vi "PELLETID.vi"(0 "NXT/EV3":T1) -> (6 "Marble ID#":i32, 7 "NXT/EV3 2":T1)   [LabVIEW 2016]
uses:
  <vilib>/NXT/Subs/LVHSConnector.ctl
  <vilib>/NXT/LegoClasses/BrickReference/BrickReference.lvclass
  <vilib>/NXT/Block Support/NXT_InputPort.ctl
  <vilib>/NXT/Dual Mode Library/Sensors/EV3_Color_RGB.vi
  <vilib>/NXT/Dual Mode Library/prims/inRangeAndCoerce/inRangeAndCoerce_int.vi
panel:
  out "RGB Color":cluster{"Red":u8, "Green":u8, "Blue":u8}
  out "Marble ID":string
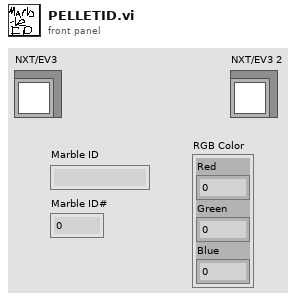
[diagram p1: front panel]
types:
  T1 = typedef "LVHSConnector.ctl" = refnum<class "BrickReference.lvclass">
  T2 = typedef "NXT_InputPort.ctl" = u32
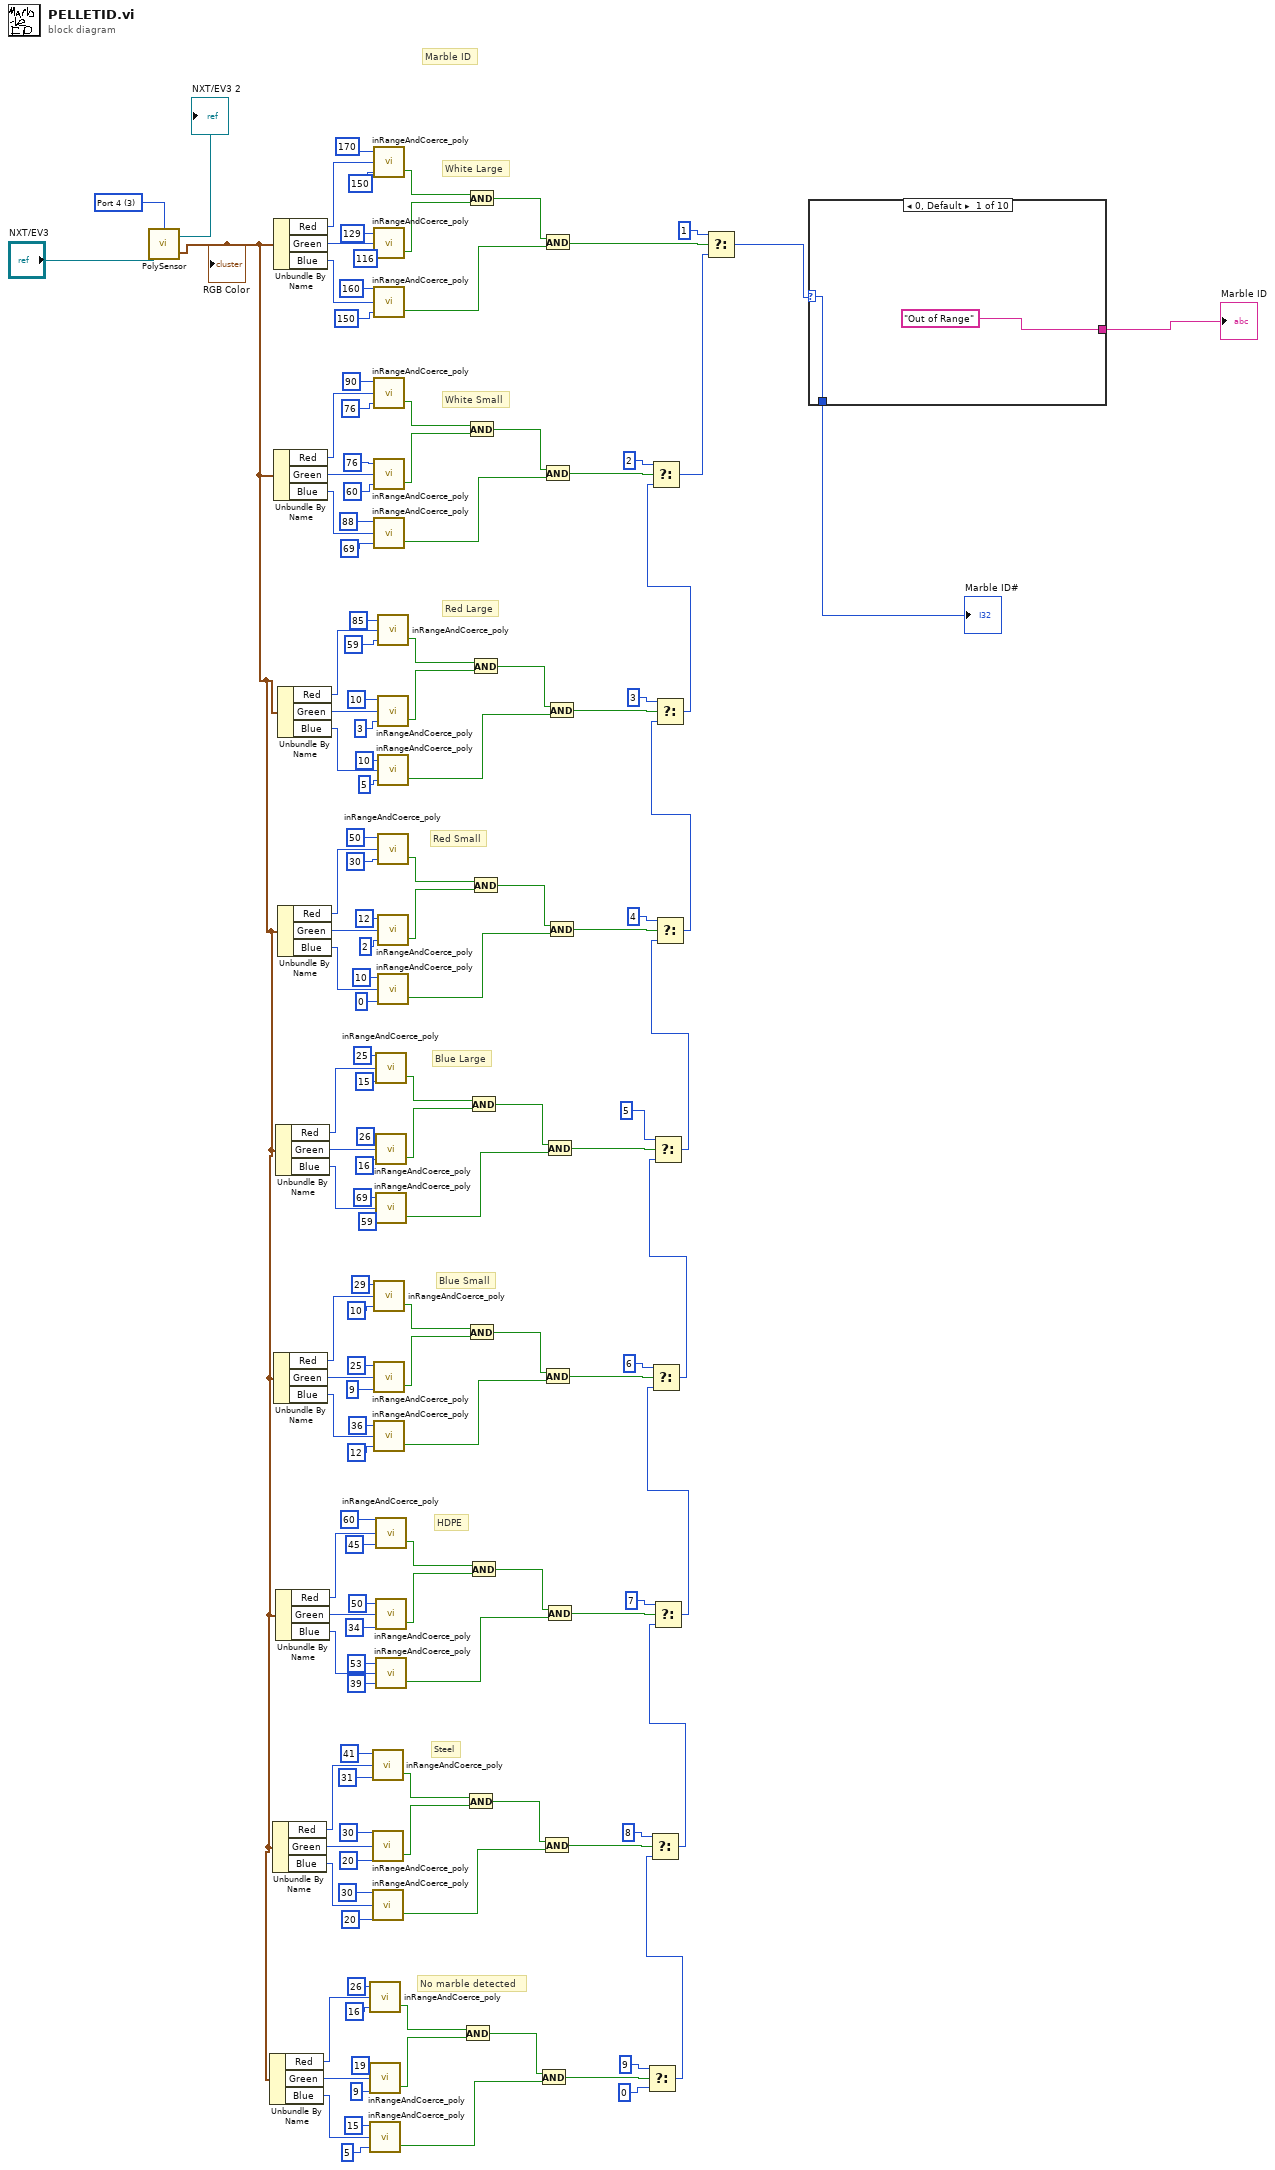
[diagram p0: block diagram]
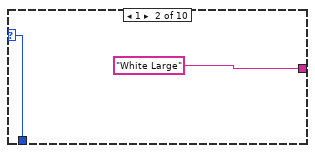
[diagram p2: hidden frame]
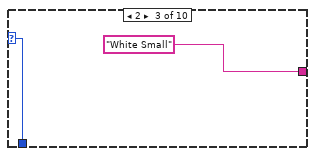
[diagram p3: hidden frame]
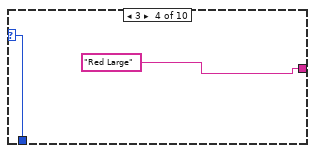
[diagram p4: hidden frame]
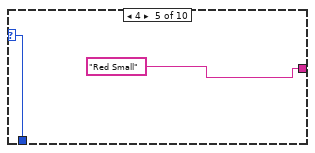
[diagram p5: hidden frame]
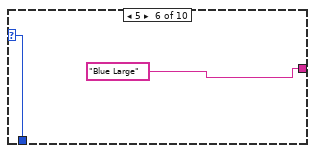
[diagram p6: hidden frame]
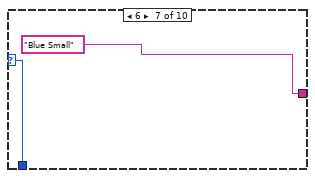
[diagram p7: hidden frame]
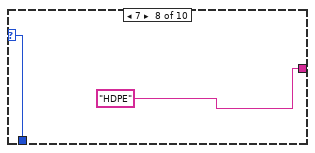
[diagram p8: hidden frame]
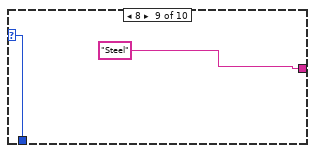
[diagram p9: hidden frame]
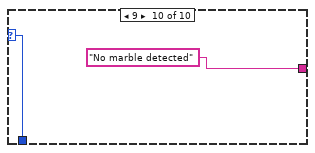
[diagram p10: hidden frame]
diagram:
  w6 = T2 3 items=["Port 1", "Port 2", "Port 3", "Port 4"] ("Port (Port 1)")
  # "No marble detected"
  # "Steel"
  # "HDPE"
  # "Blue Small"
  # "Blue Large"
  # "Red Small"
  # "Red Large"
  # "White Small"
  # "White Large"
  # "Marble ID"
  n1 = call-poly <vilib>:"PolySensor.vi"("NXT/EV3"="NXT/EV3", "Port (Port 1)"=w6) -> ("RGB Color"=w7:cluster{"Red":u8, "Green":u8, "Blue":u8}, "NXT/EV3"=→"NXT/EV3 2":T1)  [unwired: 1 in]
  "RGB Color" <- w7
  n2 = Unbundle By Name(w7) -> ("Red"=w72:u8, "Green"=w71:u8, "Blue"=w70:u8)
  n3 = Unbundle By Name(w7) -> ("Red"=w82:u8, "Green"=w81:u8, "Blue"=w80:u8)
  n4 = Unbundle By Name(w7) -> ("Red"=w151:u8, "Green"=w150:u8, "Blue"=w149:u8)
  n5 = Unbundle By Name(w7) -> ("Red"=w142:u8, "Green"=w141:u8, "Blue"=w140:u8)
  n6 = Unbundle By Name(w7) -> ("Red"=w102:u8, "Green"=w101:u8, "Blue"=w100:u8)
  n7 = Unbundle By Name(w7) -> ("Red"=w111:u8, "Green"=w110:u8, "Blue"=w1:u8)
  n8 = Unbundle By Name(w7) -> ("Red"=w92:u8, "Green"=w91:u8, "Blue"=w90:u8)
  n9 = Unbundle By Name(w7) -> ("Red"=w132:u8, "Green"=w131:u8, "Blue"=w130:u8)
  n10 = Unbundle By Name(w7) -> ("Red"=w122:u8, "Green"=w121:u8, "Blue"=w120:u8)
  n11 = call-poly <vilib>:"inRangeAndCoerce_poly.vi"("lower limit"=16, "x"=w72, "upper limit"=26) -> ("In Range?"=w69:bool)  [unwired: 1 out]
  n12 = call-poly <vilib>:"inRangeAndCoerce_poly.vi"("lower limit"=9, "x"=w71, "upper limit"=19) -> ("In Range?"=w68:bool)  [unwired: 1 out]
  n13 = call-poly <vilib>:"inRangeAndCoerce_poly.vi"("lower limit"=5, "x"=w70, "upper limit"=15) -> ("In Range?"=w66:bool)  [unwired: 1 out]
  n14 = call-poly <vilib>:"inRangeAndCoerce_poly.vi"("lower limit"=31, "x"=w82, "upper limit"=41) -> ("In Range?"=w79:bool)  [unwired: 1 out]
  n15 = call-poly <vilib>:"inRangeAndCoerce_poly.vi"("lower limit"=20, "x"=w81, "upper limit"=30) -> ("In Range?"=w78:bool)  [unwired: 1 out]
  n16 = call-poly <vilib>:"inRangeAndCoerce_poly.vi"("lower limit"=20, "x"=w80, "upper limit"=30) -> ("In Range?"=w76:bool)  [unwired: 1 out]
  n17 = call-poly <vilib>:"inRangeAndCoerce_poly.vi"("lower limit"=150, "x"=w151, "upper limit"=170) -> ("In Range?"=w148:bool)  [unwired: 1 out]
  n18 = call-poly <vilib>:"inRangeAndCoerce_poly.vi"("lower limit"=116, "x"=w150, "upper limit"=129) -> ("In Range?"=w147:bool)  [unwired: 1 out]
  n19 = call-poly <vilib>:"inRangeAndCoerce_poly.vi"("lower limit"=150, "x"=w149, "upper limit"=160) -> ("In Range?"=w145:bool)  [unwired: 1 out]
  n20 = call-poly <vilib>:"inRangeAndCoerce_poly.vi"("lower limit"=76, "x"=w142, "upper limit"=90) -> ("In Range?"=w139:bool)  [unwired: 1 out]
  n21 = call-poly <vilib>:"inRangeAndCoerce_poly.vi"("lower limit"=60, "x"=w141, "upper limit"=76) -> ("In Range?"=w138:bool)  [unwired: 1 out]
  n22 = call-poly <vilib>:"inRangeAndCoerce_poly.vi"("lower limit"=69, "x"=w140, "upper limit"=88) -> ("In Range?"=w136:bool)  [unwired: 1 out]
  n23 = call-poly <vilib>:"inRangeAndCoerce_poly.vi"("lower limit"=10, "x"=w102, "upper limit"=29) -> ("In Range?"=w99:bool)  [unwired: 1 out]
  n24 = call-poly <vilib>:"inRangeAndCoerce_poly.vi"("lower limit"=9, "x"=w101, "upper limit"=25) -> ("In Range?"=w98:bool)  [unwired: 1 out]
  n25 = call-poly <vilib>:"inRangeAndCoerce_poly.vi"("lower limit"=12, "x"=w100, "upper limit"=36) -> ("In Range?"=w96:bool)  [unwired: 1 out]
  n26 = call-poly <vilib>:"inRangeAndCoerce_poly.vi"("lower limit"=15, "x"=w111, "upper limit"=25) -> ("In Range?"=w109:bool)  [unwired: 1 out]
  n27 = call-poly <vilib>:"inRangeAndCoerce_poly.vi"("lower limit"=16, "x"=w110, "upper limit"=26) -> ("In Range?"=w108:bool)  [unwired: 1 out]
  n28 = call-poly <vilib>:"inRangeAndCoerce_poly.vi"("lower limit"=59, "x"=w1, "upper limit"=69) -> ("In Range?"=w106:bool)  [unwired: 1 out]
  n29 = call-poly <vilib>:"inRangeAndCoerce_poly.vi"("lower limit"=45, "x"=w92, "upper limit"=60) -> ("In Range?"=w89:bool)  [unwired: 1 out]
  n30 = call-poly <vilib>:"inRangeAndCoerce_poly.vi"("lower limit"=34, "x"=w91, "upper limit"=50) -> ("In Range?"=w88:bool)  [unwired: 1 out]
  n31 = call-poly <vilib>:"inRangeAndCoerce_poly.vi"("lower limit"=39, "x"=w90, "upper limit"=53) -> ("In Range?"=w86:bool)  [unwired: 1 out]
  n32 = call-poly <vilib>:"inRangeAndCoerce_poly.vi"("lower limit"=59, "x"=w132, "upper limit"=85) -> ("In Range?"=w129:bool)  [unwired: 1 out]
  n33 = call-poly <vilib>:"inRangeAndCoerce_poly.vi"("lower limit"=3, "x"=w131, "upper limit"=10) -> ("In Range?"=w128:bool)  [unwired: 1 out]
  n34 = call-poly <vilib>:"inRangeAndCoerce_poly.vi"("lower limit"=5, "x"=w130, "upper limit"=10) -> ("In Range?"=w126:bool)  [unwired: 1 out]
  n35 = call-poly <vilib>:"inRangeAndCoerce_poly.vi"("lower limit"=30, "x"=w122, "upper limit"=50) -> ("In Range?"=w119:bool)  [unwired: 1 out]
  n36 = call-poly <vilib>:"inRangeAndCoerce_poly.vi"("lower limit"=2, "x"=w121, "upper limit"=12) -> ("In Range?"=w118:bool)  [unwired: 1 out]
  n37 = call-poly <vilib>:"inRangeAndCoerce_poly.vi"("lower limit"=0, "x"=w120, "upper limit"=10) -> ("In Range?"=w116:bool)  [unwired: 1 out]
  n38 = And(x=w69, y=w68) -> (x .and. y?=w67:bool)
  n39 = And(x=w79, y=w78) -> (x .and. y?=w77:bool)
  n40 = And(x=w148, y=w147) -> (x .and. y?=w146:bool)
  n41 = And(x=w139, y=w138) -> (x .and. y?=w137:bool)
  n42 = And(x=w99, y=w98) -> (x .and. y?=w97:bool)
  n43 = And(x=w109, y=w108) -> (x .and. y?=w107:bool)
  n44 = And(x=w89, y=w88) -> (x .and. y?=w87:bool)
  n45 = And(x=w129, y=w128) -> (x .and. y?=w127:bool)
  n46 = And(x=w119, y=w118) -> (x .and. y?=w117:bool)
  n47 = And(x=w67, y=w66) -> (x .and. y?=w65:bool)
  n48 = And(x=w77, y=w76) -> (x .and. y?=w75:bool)
  n49 = And(x=w146, y=w145) -> (x .and. y?=w144:bool)
  n50 = And(x=w137, y=w136) -> (x .and. y?=w135:bool)
  n51 = And(x=w97, y=w96) -> (x .and. y?=w95:bool)
  n52 = And(x=w107, y=w106) -> (x .and. y?=w105:bool)
  n53 = And(x=w87, y=w86) -> (x .and. y?=w85:bool)
  n54 = And(x=w127, y=w126) -> (x .and. y?=w125:bool)
  n55 = And(x=w117, y=w116) -> (x .and. y?=w115:bool)
  n56 = Select(t=9, s=w65, f=0) -> (s? t:f=w63:i32)
  n57 = Select(t=8, s=w75, f=w63) -> (s? t:f=w73:i32)
  n58 = Select(t=7, s=w85, f=w73) -> (s? t:f=w83:i32)
  n59 = Select(t=6, s=w95, f=w83) -> (s? t:f=w93:i32)
  n60 = Select(t=5, s=w105, f=w93) -> (s? t:f=w103:i32)
  n61 = Select(t=4, s=w115, f=w103) -> (s? t:f=w112:i32)
  n62 = Select(t=3, s=w125, f=w112) -> (s? t:f=w113:i32)
  n63 = Select(t=2, s=w135, f=w113) -> (s? t:f=w133:i32)
  n64 = Select(t=1, s=w144, f=w133) -> (s? t:f=w3:i32)
  n65 = case shown="0, Default" w3 {
    selector: w3 -> [w152 w154 w156 w158 w160 w162 w164 w166 w168 w170]
    tunnel: ["Out of Range" "White Large" "White Small" "Red Large" "Red Small" "Blue Large" "Blue Small" "HDPE" "Steel" "No marble detected"] -> w123
    tunnel: [w152 w154 w156 w158 w160 w162 w164 w166 w168 w170] -> w2
    frame 0, Default {
    }
    frame 1 {
    }
    frame 2 {
    }
    frame 3 {
    }
    frame 4 {
    }
    frame 5 {
    }
    frame 6 {
    }
    frame 7 {
    }
    frame 8 {
    }
    frame 9 {
    }
  }
  "Marble ID" <- w123
  "Marble ID#" <- w2
